vi "Save As FITS.vi"(10 "typ":i32, 11 "szFileTitle":string) -> (2 "function return":u32, 3 "szFileTitle out":string)   [LabVIEW 2018, in "AndorSDK.lvlib"]
doc: "EXPNETTYPE unsigned int WINAPI SaveAsFITS(char * szFileTitle, int typ);"
uses:
  AndorSDK.lvlib
  ATMCD32D.dll
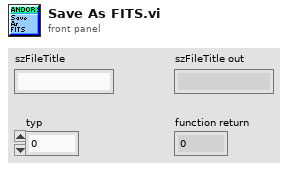
[diagram p1: front panel]
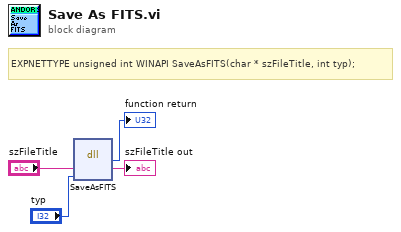
[diagram p0: block diagram]
diagram:
  # "EXPNETTYPE unsigned int WINAPI SaveAsFITS(char * szFileTitle, int typ);"
  n1 = dll-call lib="PTH2babs E\nPersönliches02 - Arbeit03-HiwijobsLabviewCodelibANDOR\tAndor SDK\nATMCD32D.*" fn="SaveAsFITS"("szFileTitle"="szFileTitle", "typ"="typ") -> (→"function return":u32, "szFileTitle"=→"szFileTitle out":string)  [unwired: 4 in, 2 out]
